vi "Script_Selector.vi"(11 "Standard":T1(ring)) -> (3 "Script":string)   [LabVIEW 2014]
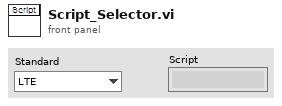
[diagram p1: front panel]
types:
  T1 = enum16{"LTE", "WCDMA", "GSM", "EDGE", "CW", "CWM"}
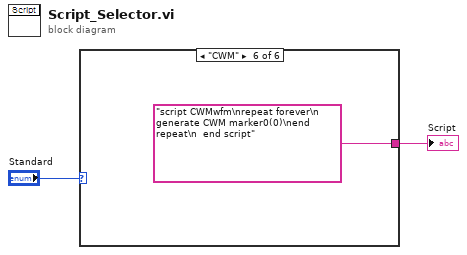
[diagram p0: block diagram]
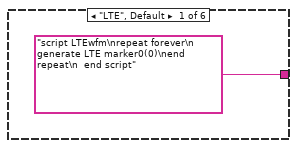
[diagram p2: hidden frame]
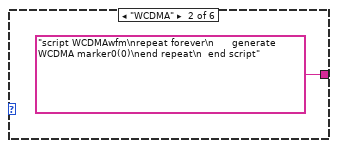
[diagram p3: hidden frame]
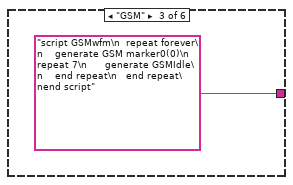
[diagram p4: hidden frame]
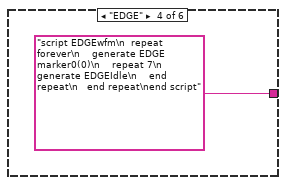
[diagram p5: hidden frame]
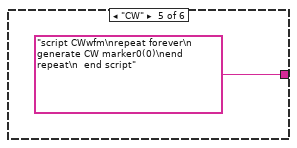
[diagram p6: hidden frame]
diagram:
  n1 = case shown="\"CWM\"" "Standard" {
    tunnel: ["script LTEwfm\nrepeat forever\n      generate LTE marker0(0)\nend repeat\n  end script" "script WCDMAwfm\nrepeat forever\n      generate WCDMA marker0(0)\nend repeat\n  end script" "script GSMwfm\n  repeat forever\n    generate GSM marker0(0)\n    repeat 7\n      generate GSMIdle\n    end repeat\n   end repeat\nend script" "script EDGEwfm\n  repeat forever\n    generate EDGE marker0(0)\n    repeat 7\n      generate EDGEIdle\n    end repeat\n   end repeat\nend script" "script CWwfm\nrepeat forever\n      generate CW marker0(0)\nend repeat\n  end script" "script CWMwfm\nrepeat forever\n      generate CWM marker0(0)\nend repeat\n  end script"] -> w2
    frame "LTE", Default {
    }
    frame "WCDMA" {
    }
    frame "GSM" {
    }
    frame "EDGE" {
    }
    frame "CW" {
    }
    frame "CWM" {
    }
  }
  "Script" <- w2
